vi "Terminal-Alert-GearSystem.vi"(11 "齿轮子系统设备信息":T1) -> (3 "齿轮子系统设备信息输出":T1)   [LabVIEW 2014]
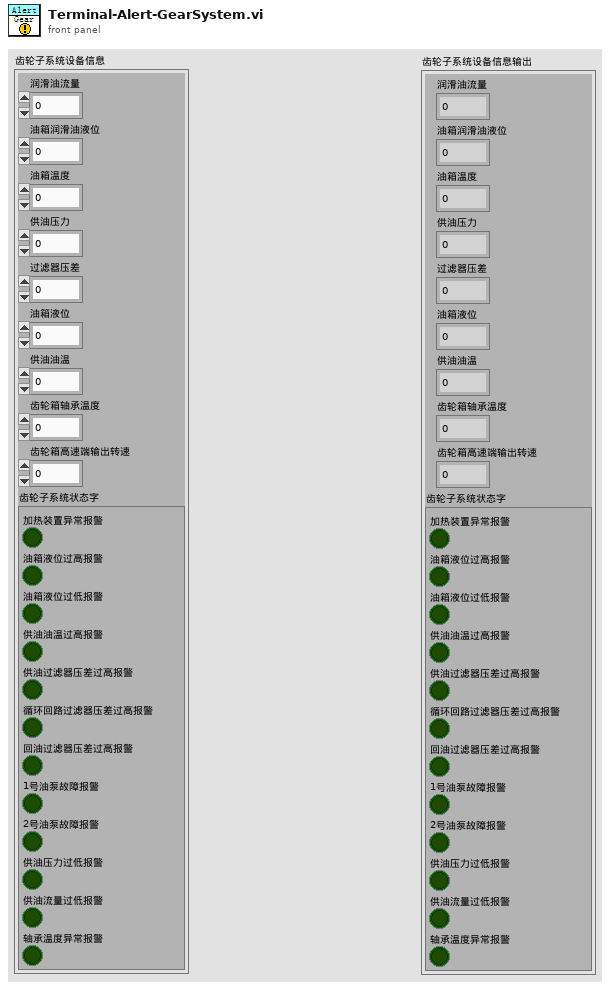
[diagram p1: front panel]
types:
  T1 = cluster{"润滑油流量":u16, "油箱润滑油液位":u16, "油箱温度":u16, "供油压力":u16, "过滤器压差":u16, "油箱液位":u16, "供油油温":u16, "齿轮箱轴承温度":u16, "齿轮箱高速端输出转速":u16, "齿轮子系统状态字":cluster{"加热装置异常报警":bool, "油箱液位过高报警":bool, "油箱液位过低报警":bool, "供油油温过高报警":bool, "供油过滤器压差过高报警":bool, "循环回路过滤器压差过高报警":bool, "回油过滤器压差过高报警":bool, "1号油泵故障报警":bool, "2号油泵故障报警":bool, "供油压力过低报警":bool, "供油流量过低报警":bool, "轴承温度异常报警":bool}}
  T2 = cluster{"报警级别":string, "报警系统":string, "报警详情":string, "备注":string}
  T3 = cluster{"加热装置异常报警":bool, "油箱液位过高报警":bool, "油箱液位过低报警":bool, "供油油温过高报警":bool, "供油过滤器压差过高报警":bool, "循环回路过滤器压差过高报警":bool, "回油过滤器压差过高报警":bool, "1号油泵故障报警":bool, "2号油泵故障报警":bool, "供油压力过低报警":bool, "供油流量过低报警":bool, "轴承温度异常报警":bool}
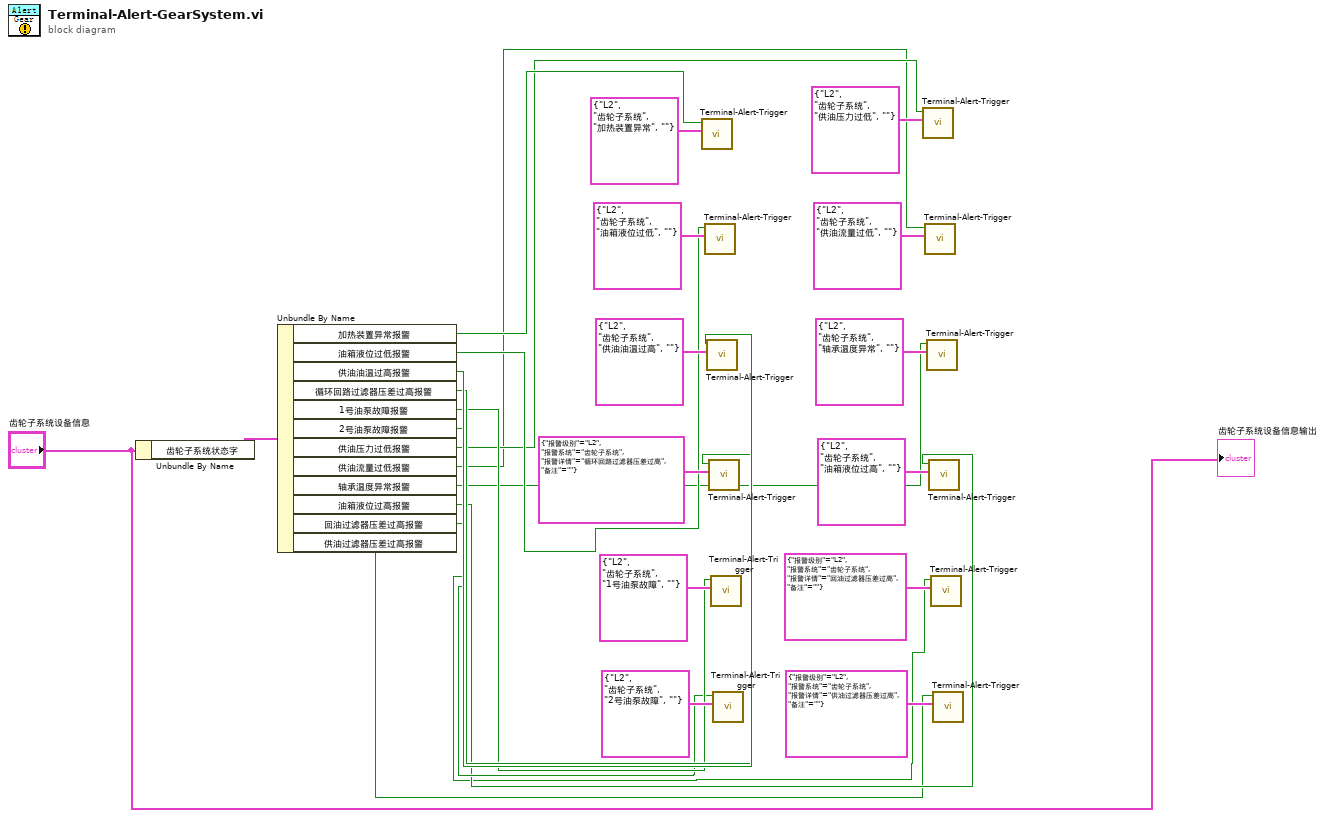
[diagram p0: block diagram]
diagram:
  n1 = Unbundle By Name("齿轮子系统设备信息") -> ("齿轮子系统状态字"=w26:T3)
  n2 = Unbundle By Name(w26) -> ("加热装置异常报警"=w13:bool, "油箱液位过低报警"=w12:bool, "供油油温过高报警"=w11:bool, "循环回路过滤器压差过高报警"=w10:bool, "1号油泵故障报警"=w9:bool, "2号油泵故障报警"=w8:bool, "供油压力过低报警"=w7:bool, "供油流量过低报警"=w6:bool, "轴承温度异常报警"=w5:bool, "油箱液位过高报警"=w4:bool, "回油过滤器压差过高报警"=w3:bool, "供油过滤器压差过高报警"=w2:bool)
  n3 = call "Terminal-Alert-Trigger.vi"("报警信息"=T2 {"报警级别"="L2", "报警系统"="齿轮子系统", "报警详情"="加热装置异常", "备注"=""}, "是否触发(T)"=w13) -> ()  [unwired: 9 in, 1 out]
  n4 = call "Terminal-Alert-Trigger.vi"("报警信息"=T2 {"报警级别"="L2", "报警系统"="齿轮子系统", "报警详情"="油箱液位过低", "备注"=""}, "是否触发(T)"=w12) -> ()  [unwired: 9 in, 1 out]
  n5 = call "Terminal-Alert-Trigger.vi"("报警信息"=T2 {"报警级别"="L2", "报警系统"="齿轮子系统", "报警详情"="供油油温过高", "备注"=""}, "是否触发(T)"=w11) -> ()  [unwired: 9 in, 1 out]
  n6 = call "Terminal-Alert-Trigger.vi"("报警信息"=T2 {"报警级别"="L2", "报警系统"="齿轮子系统", "报警详情"="循环回路过滤器压差过高", "备注"=""}, "是否触发(T)"=w10) -> ()  [unwired: 9 in, 1 out]
  n7 = call "Terminal-Alert-Trigger.vi"("报警信息"=T2 {"报警级别"="L2", "报警系统"="齿轮子系统", "报警详情"="1号油泵故障", "备注"=""}, "是否触发(T)"=w9) -> ()  [unwired: 9 in, 1 out]
  n8 = call "Terminal-Alert-Trigger.vi"("报警信息"=T2 {"报警级别"="L2", "报警系统"="齿轮子系统", "报警详情"="2号油泵故障", "备注"=""}, "是否触发(T)"=w8) -> ()  [unwired: 9 in, 1 out]
  n9 = call "Terminal-Alert-Trigger.vi"("报警信息"=T2 {"报警级别"="L2", "报警系统"="齿轮子系统", "报警详情"="供油压力过低", "备注"=""}, "是否触发(T)"=w7) -> ()  [unwired: 9 in, 1 out]
  n10 = call "Terminal-Alert-Trigger.vi"("报警信息"=T2 {"报警级别"="L2", "报警系统"="齿轮子系统", "报警详情"="供油流量过低", "备注"=""}, "是否触发(T)"=w6) -> ()  [unwired: 9 in, 1 out]
  n11 = call "Terminal-Alert-Trigger.vi"("报警信息"=T2 {"报警级别"="L2", "报警系统"="齿轮子系统", "报警详情"="轴承温度异常", "备注"=""}, "是否触发(T)"=w5) -> ()  [unwired: 9 in, 1 out]
  n12 = call "Terminal-Alert-Trigger.vi"("报警信息"=T2 {"报警级别"="L2", "报警系统"="齿轮子系统", "报警详情"="油箱液位过高", "备注"=""}, "是否触发(T)"=w4) -> ()  [unwired: 9 in, 1 out]
  n13 = call "Terminal-Alert-Trigger.vi"("报警信息"=T2 {"报警级别"="L2", "报警系统"="齿轮子系统", "报警详情"="回油过滤器压差过高", "备注"=""}, "是否触发(T)"=w3) -> ()  [unwired: 9 in, 1 out]
  n14 = call "Terminal-Alert-Trigger.vi"("报警信息"=T2 {"报警级别"="L2", "报警系统"="齿轮子系统", "报警详情"="供油过滤器压差过高", "备注"=""}, "是否触发(T)"=w2) -> ()  [unwired: 9 in, 1 out]
  "齿轮子系统设备信息输出" <- "齿轮子系统设备信息"
